vi "Rename Library.vi"(6 "Rename Library File Path":path, 8 "error in":errorcluster, 9 "Name Library File Path":path, 10 "Active Project":refnum<vi>) -> (0 "error out":errorcluster, 2 "Library Ref":refnum<vi>)   [LabVIEW 2020, in "_Rename.lvlib" / "_Rename.lvclass"]
uses:
  _Rename.lvclass
  <vilib>/Utility/EditLVLibs/Edit LVLibs.lvlib
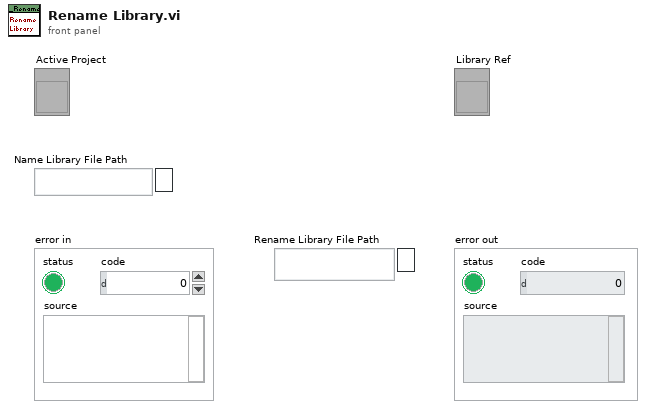
[diagram p1: front panel]
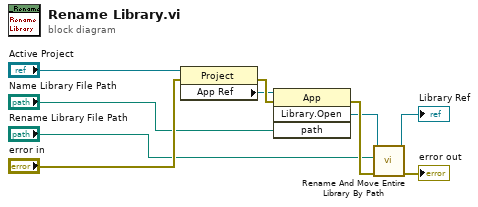
[diagram p0: block diagram]
diagram:
  n1 = property class="Project"(reference="Active Project", error in="error in") -> (error out=w8:errorcluster, "App Ref"=w7:refnum<vi>)  [unwired: 1 out]
  n2 = invoke class="App" method="Library.Open"(reference=w7, error in=w8, "path"="Name Library File Path") -> (error out=w9:errorcluster, "Open Library"=w2:refnum<vi>)  [unwired: 1 in, 2 out]
  n3 = call <vilib>:"Rename And Move Entire Library By Path.vi"("error in (no error)"=w9, "New library path"="Rename Library File Path", "Library ref in"=w2) -> ("error out"=→"error out":errorcluster, "Library ref out"=→"Library Ref":refnum<vi>)  [unwired: 7 in]
